vi "LSMcontroller_v59_PIzstage.vi"() -> ()   [LabVIEW 2015] (continued)
                                }
                                frame 5..7 {
                                n2125 = Index Array(array=w5021, index=0) -> (element=w5022:T19)
                                n2126 = call "waveformparamsv2.vi"("command"="get") -> ("Params out"=w5027:T15)  [unwired: 4 in, 2 out]
                                n2127 = in-place {
                                in-place-border: w5024 -> [w5031]
                                in-place-border: w5022 -> [w5029]
                                n2128 = in-place-cluster #43(w5027) -> ("DO parameters"=w5032:T18)
                                n2129 = in-place {
                                in-place-border: w5029 -> [w5033]
                                n2130 = in-place-array #44(w5032, w5031) -> ()  [unwired: 1 out]
                                n2131 = in-place-array #44(w5033) -> (w5030:T18)  [unwired: 1 out]
                                }
                                n2132 = in-place-cluster #43("DO parameters"=w5030) -> (w5025:T15)
                                }
                                n2133 = call "waveformparamsv2.vi"("command"="set", "Params in"=w5025) -> ()  [unwired: 3 in, 3 out]
                                }
                                }
                                }
                                frame #2 {
                                n2134 = local read "Measurement"() -> (w5035:T4)
                                n2135 = To Unsigned Long Integer(number=w5035) -> (unsigned 32bit integer=w5034:u32)
                                n2136 = case shown="5..7" w5034 {
                                tunnel: w5037 -> [_ w5041]
                                tunnel: w5036 -> [_ w5039]
                                frame 0..4, Default {
                                }
                                frame 5..7 {
                                n2137 = Index Array(array=w5039, index=0) -> (element=w5038:digitalwaveform)
                                n2138 = call "waveformsDObuffer.vi"("command"="get") -> ("DO wf out"=w5043:digitalwaveform[])  [unwired: 1 in]
                                n2139 = Replace Array Subset(array=w5043, new element=w5038, index=w5041) -> (w5045:digitalwaveform[])
                                n2140 = call "waveformsDObuffer.vi"("DO wf in"=w5045, "command"="set") -> ()  [unwired: 1 out]
                                }
                                }
                                }
                                }
                                }
                                }
                              }
                              frame #4 {
                                n2141 = call "Used AO lines.vi"() -> ("used AO names"=w5048:string[], "used AO lines"=w5046:tag[])  [unwired: 2 in]
                                n2142 = control-ref of="Analog Lines Plot"() -> (w5047:refnum<vi>)
                                n2143 = control-ref of="Digital Lines Plot"() -> (w5049:refnum<vi>)
                                n2144 = call "Used DO lines.vi"() -> ("used DO names"=w5050:string[], "used DO lines"=w5051:tag[])  [unwired: 2 in]
                                n2145 = local write "Analog Used Lines"(w5046) -> ()
                                n2146 = local write "Analog Used Names"(w5048) -> ()
                                n2147 = local write "Digital Used Lines"(w5051) -> ()
                                n2148 = local write "Digital Used Names"(w5050) -> ()
                                n2149 = call "prepDOWaveplot.vi"("DigitalGraph in"=w5049, "used DO names"=w5050) -> ()  [unwired: 1 in]
                                n2150 = call "prepAOWaveplot.vi"("WaveformGraph in"=w5047, "Analog Used Names"=w5048) -> ()  [unwired: 1 in]
                              }
                              frame #5 {
                                n2151 = local read "Meastab"() -> (w5066:enum32{"X-Y Image", "Linescan", "Timetrace"})
                                n2152 = property on="refwf" class="Ring (strict)"() -> ("RingText.Text"=w5063:string)  [unwired: 2 in, 2 out]
                                n2153 = case shown="\"Timetrace\"" w5066 {
                                tunnel: [w5068 w5069] -> w5067
                                frame "X-Y Image", Default {
                                n2154 = local read "Sampling rate"() -> (w5068:dbl)
                                }
                                frame "Timetrace" {
                                n2155 = local read "srateAODOtt"() -> (w5069:dbl)
                                }
                                }
                                n2156 = call "waveformsAObuffer.vi"("command"="get") -> ("AO wf out"=w5054:waveform(dbl)[])  [unwired: 1 in]
                                n2157 = local read "wavdet"() -> (w5064:bool)
                                n2158 = call "waveformsDObuffer.vi"("command"="get") -> ("DO wf out"=w5058:digitalwaveform[])  [unwired: 1 in]
                                n2159 = call "correctwaveformsizetemp.vi"("new sampling frequency (Hz)"=w5067, "start"=FALSE, "reference waveforms to"=w5063, "Analog waveforms in"=w5054, "stop"=TRUE, "Digital waveforms in"=w5058) -> ("analog wf out"=w5060:waveform(dbl)[], "Digital wf out"=w5062:digitalwaveform[], "measpoints"=w5065:i32)
                                n2160 = local write "Analog Lines Plot"(w5060) -> ()
                                n2161 = call "GetNumCamFramesv2.vi"("Digital Waveform Graph"=w5062) -> ("Numeric"=w5061:i32)  [unwired: 10 in]
                                n2162 = local write "Digital Lines Plot"(w5062) -> ()
                                n2163 = call "waveformsDObuffer.vi"("DO wf in"=w5062, "command"="set") -> ()  [unwired: 1 out]
                                n2164 = call "waveformsAObuffer.vi"("AO wf in"=w5060, "command"="set") -> ()  [unwired: 1 out]
                                n2165 = local write "Total Camera Frames"(w5061) -> ()
                                n2166 = case shown="True" w5064 {
                                tunnel: w5065 -> [_ w5070]
                                frame False {
                                }
                                frame True {
                                n2167 = local write "# of frames"(w5070) -> ()
                                }
                                }
                              }
                            }
                            n2168 = call "stoperaseCI.vi"() -> ()  [unwired: 12 in]
                            n2169 = call "stoperaseDO_img.vi"() -> ()  [unwired: 12 in]
                            n2170 = call "stoperaseAO_img.vi"() -> ()  [unwired: 12 in]
                            n2171 = call "stoperaseAI_img.vi"() -> ()  [unwired: 12 in]
                          }
                          frame #9 {
                            w5080 = FALSE ("Value (Signaling)")
                            n2172 = local read "save\ndata"() -> (w5075:bool)
                            n2173 = case shown="True" w5075 {
                              tunnel: w5074 -> [_ w5087]
                              frame False {
                              }
                              frame True {
                                n2174 = call "closebinaryfiles.vi"() -> ()  [unwired: 12 in]
                                n2175 = local read "filename prefix"() -> (w5089:string)
                                n2176 = local read "data dir"() -> (w5088:path)
                                n2177 = call "saveparams.vi"("timestamp"=w5087, "filename prefix in"=w5089, "data dir in"=w5088) -> ()  [unwired: 1 in]
                              }
                            }
                            n2178 = call "2pparameters.vi"("command"="get") -> ("params out"=w5071:T11)  [unwired: 1 in]
                            n2179 = Unbundle By Name(w5071) -> ("auto OD"=w5072:bool)
                            n2180 = case shown="True" w5072 {
                              frame False {
                              }
                              frame True {
                                n2181 = call "configuration.vi"("command"="get") -> ("config out"=w5083:T12)  [unwired: 2 in, 1 out]
                                n2182 = call "2pparameters.vi"("command"="get") -> ("params out"=w5086:T11)  [unwired: 1 in]
                                n2183 = Unbundle By Name(w5083) -> ("contour OD"=w5081:u16)
                                n2184 = Unbundle By Name(w5086) -> ("ODfilt"=w5082:u16)
                                n2185 = call "filterwheelcontrol_nothorlabslib.vi"("Current OD filt"=w5081, "New ODfilt"=w5082) -> ()  [unwired: 1 in]
                              }
                            }
                            n2186 = property on="Start" class="Bool (strict)"("Val(Sgnl)"=w5080) -> ()  [unwired: 2 in, 2 out]
                            n2187 = property on="Start" class="Bool (strict)"("Visible"=TRUE, "DisabledEnum"=T7."Enabled" ("Disabled")) -> ()  [unwired: 2 in, 2 out]
                            n2188 = property on="Stop" class="Bool (strict)"("Val(Sgnl)"=w5080) -> ()  [unwired: 2 in, 2 out]
                            n2189 = property on="Stop" class="Bool (strict)"("Visible"=FALSE, "DisabledEnum"=T7."Disabled" ("Disabled")) -> ()  [unwired: 2 in, 2 out]
                          }
                          frame #10 {
                            w5092 = T22 2 items=["no dialog", "OK message", "continue or stop message", "OK message + warnings", "continue/stop + warnings"] ("type of dialog (OK msg:1)")
                            n2190 = call "displayerrors.vi"() -> ("error IO"=w5093:errorcluster)
                            n2191 = call <vilib>:"General Error Handler.vi"("type of dialog (OK msg:1)"=w5092, "error in (no error)"=w5093) -> ("error out"=w5091:errorcluster)  [unwired: 9 in, 4 out]
                            n2192 = call <vilib>:"Clear Errors.vi"("error in (no error)"=w5091) -> ("error out"=w5090:errorcluster)  [unwired: 5 in, 1 out]
                            n2193 = call "seterrors.vi"("error IO"=w5090) -> ()
                          }
                        }
                      }
                    }
                  }
                  frame "Lifetime (point)" {
                    # "Disabled for conversion to 64 bit"
                    n2194 = disable-structure shown="Disabled" {
                      frame Disabled {
                        n2195 = stacked-sequence {
                          frame #0 {
                            w5104 = 12.5 ("x")
                            # "get from syncrate"
                            n2196 = local read "Bin size"() -> (w5098:T6)
                            n2197 = local read "Vx-ref"() -> (w5110:dbl)
                            n2198 = local read "Vy-ref"() -> (w5111:dbl)
                            n2199 = call "2pparameters.vi"("command"="get") -> ("params out"=w5096:T11)  [unwired: 1 in]
                            n2200 = Scale By Power Of 2(n=w5098, x=1.0 ("Y Scale.Range:Minimum")) -> (x*2^n=w5107:dbl)
                            n2201 = call "setposition.vi"("Vy"=w5111, "Vx"=w5110) -> ()  [unwired: 1 in]
                            n2202 = Unbundle By Name(w5096) -> ("autoshutter"=w5097:bool)
                            n2203 = Multiply(x=3000.0 ("Y Scale.Range:Minimum"), y=w5107) -> (x*y=w5105:dbl)
                            n2204 = Compound Arithmetic op=MULTIPLY(w5104, invert 3200.0 ("X Scale.Offset and Multiplier:Multiplier"), w5107) -> (w5106:dbl)
                            n2205 = case shown="True" w5097 {
                              frame False {
                              }
                              frame True {
                                n2206 = call "shuttercontrol.vi"("command"="open") -> ()  [unwired: 1 in, 1 out]
                              }
                            }
                            n2207 = call "lifetimeparameters.vi"("command"="get") -> ("Params out"=w5102:T20)  [unwired: 1 in]
                            n2208 = property on="Histogram" class="WFGraph (strict)"("XScale.Maximum"=w5104, "XScale.Minimum"=0.0 ("X Scale.Range:Minimum"), "YScale.Maximum"=w5105, "YScale.Minimum"=0.1 ("Y Scale.Range:Minimum"), "XScale.Multiplier"=w5106) -> ()  [unwired: 2 in, 2 out]
                            n2209 = Bundle By Name(cluster=w5102, "Bin size"=w5098) -> (w5103:T20)
                            n2210 = call "lifetimeparameters.vi"("Params in"=w5103, "command"="set") -> ()  [unwired: 1 out]
                            n2211 = property on="Histogram 2" class="WFGraph (strict)"("YScale.Maximum"=w5105, "XScale.Multiplier"=w5106, "XScale.Maximum"=w5104) -> ()  [unwired: 2 in, 2 out]
                            n2212 = call "2pparameters.vi"("command"="get") -> ("params out"=w5118:T11)  [unwired: 1 in]
                            n2213 = Bundle By Name(cluster=w5118, "type"="Lifetime (point)") -> (w5116:T11)
                            n2214 = property on="Stop" class="Bool (strict)"("Visible"=TRUE, "DisabledEnum"=T7."Enabled" ("Disabled")) -> ()  [unwired: 2 in, 2 out]
                            n2215 = property on="Start" class="Bool (strict)"("Visible"=FALSE, "DisabledEnum"=T7."Disabled and Grayed Out" ("Disabled")) -> ()  [unwired: 2 in, 2 out]
                            n2216 = call "2pparameters.vi"("Params in"=w5116, "command"="set") -> ()  [unwired: 1 out]
                          }
                          frame #1 {
                            n2217 = call "setup.vi"() -> ()  [unwired: 1 in]
                          }
                          frame #2 {
                            # "main loop"
                            n2218 = call "lifetimeparameters.vi"("command"="get") -> ("Params out"=w5128:T20)  [unwired: 1 in]
                            n2219 = Unbundle By Name(w5128) -> ("devidx"=w5126:i32)
                            n2220 = for {
                              N: 10000 -> [_]
                              tunnel: [w5129] -> w5124 mode=indexing
                              i -> [w5129]
                            }
                            n2221 = while {
                              tunnel: w5126 -> [w5133]
                              tunnel: w5124 -> [w5130]
                              i -> [w5131]
                              stop <- w5135 stop-if-true
                              n2222 = Increment(x=w5131) -> (x+1=w5132:i32)
                              n2223 = dll-call lib="phlib.dll" fn="_PH_GetCountRate@8" label="PH_GetCountRate"("devidx"=w5133, "channel"=0) -> (w5134:i32)  [unwired: 5 in, 2 out]
                              "SyncRate" <- w5134
                              n2224 = stacked-sequence {
                                seq-local: [_ _ w5142 _ _] -> [_ _ _ w5155 _]
                                seq-local: [_ _ w5141 _ _] -> [_ _ _ w5154 _]
                                seq-local: [_ w5139 _ _ _] -> [_ _ w5143 _ _]
                                tunnel: w5134 -> [_ _ _ w5162 _]
                                tunnel: w5130 -> [_ _ _ w5152 _]
                                frame #0 {
                                n2225 = call "start_binned.vi"() -> ()  [unwired: 1 in]
                                }
                                frame #1 {
                                n2226 = call "get-histogram.vi"() -> ("IntegralCount"=→"Integral count":u32, "Histogram"=w5139:u32[])
                                "Histogram" <- w5139
                                }
                                frame #2 {
                                n2227 = Search 1D Array(1D array=w5143, element=u32 0) -> (index of element=w5141:i32)  [unwired: 1 in]
                                n2228 = Multiply(x=w5141, y=0.99) -> (x*y=w5147:dbl)
                                n2229 = Array Subset(array=w5143, index=0, length=w5147) -> (w5150:u32[])
                                n2230 = Array Max & Min(array=w5150) -> (max index (indices)=w5144:i32)  [unwired: 3 out]
                                n2231 = Split 1D Array(array=w5150, index=w5144) -> (second subarray=w5146:u32[])  [unwired: 1 out]
                                n2232 = Array Max & Min(array=w5146) -> (min index (indices)=w5145:i32)  [unwired: 3 out]
                                n2233 = Split 1D Array(array=w5146, index=w5145) -> (first subarray=w5142:u32[])  [unwired: 1 out]
                                "Histogram 2" <- w5142
                                }
                                frame #3 {
                                n2234 = Array Size(array=w5155) -> (size(s)=w5157:i32)
                                n2235 = Array Subset(array=w5152, index=0, length=w5157) -> (w5156:i32[])
                                n2236 = Compound Arithmetic op=MULTIPLY(1000000000.0 ("value"), invert w5162, invert w5154, w5156) -> (w5153:dbl[])
                                n2237 = call <vilib>:"Exponential Fit.vi"("Y"=w5155, "X"=w5153) -> ("damping"=w5159:dbl)  [unwired: 8 in, 5 out]
                                n2238 = Divide(x=-1.0 ("y"), y=w5159) -> (x/y=→"Lifetime (ns)":dbl)
                                }
                                frame #4 {
                                n2239 = local read "downright"() -> (w5169:bool)
                                n2240 = local read "downleft"() -> (w5171:bool)
                                n2241 = local read "upright"() -> (w5167:bool)
                                n2242 = local read "upleft"() -> (w5165:bool)
                                n2243 = local read "down"() -> (w5170:bool)
                                n2244 = local read "right"() -> (w5168:bool)
                                n2245 = local read "left"() -> (w5172:bool)
                                n2246 = local read "up"() -> (w5166:bool)
                                n2247 = Compound Arithmetic op=OR(w5165, w5166, w5167, w5168, w5169, w5170, w5171, w5172) -> (w5164:bool)
                                n2248 = case shown="True" w5164 {
                                frame False {
                                }
                                frame True {
                                n2249 = stacked-sequence {
                                frame #0 {
                                n2250 = local read "downright"() -> (w5174:bool)
                                n2251 = local read "downleft"() -> (w5176:bool)
                                n2252 = local read "BigSmall"() -> (w5173:bool)
                                n2253 = local read "upright"() -> (w5178:bool)
                                n2254 = local read "upleft"() -> (w5181:bool)
                                n2255 = local read "down"() -> (w5177:bool)
                                n2256 = local read "right"() -> (w5179:bool)
                                n2257 = local read "left"() -> (w5175:bool)
                                n2258 = local read "up"() -> (w5180:bool)
                                n2259 = call "movestageparams.vi"("command"="get") -> ("Params out"=w5184:T21)  [unwired: 1 in]
                                n2260 = Bundle By Name(cluster=w5184, "upleft"=w5181, "up"=w5180, "upright"=w5178, "right"=w5179, "downright"=w5174, "down"=w5177, "downleft"=w5176, "left"=w5175, "Bigsmall"=w5173) -> (w5185:T21)
                                n2261 = call "movestageparams.vi"("Params in"=w5185, "command"="set") -> ()  [unwired: 1 out]
                                }
                                frame #1 {
                                n2262 = call "movestage.vi"() -> ()  [unwired: 12 in]
                                }
                                frame #2 {
                                w5186 = FALSE ("OK Button")
                                w5187 = FALSE ("OK Button")
                                n2263 = property on="down" class="Bool (strict)"("Value"=w5187) -> ()  [unwired: 2 in, 2 out]
                                n2264 = property on="up" class="Bool (strict)"("Value"=w5187) -> ()  [unwired: 2 in, 2 out]
                                n2265 = property on="right" class="Bool (strict)"("Value"=w5187) -> ()  [unwired: 2 in, 2 out]
                                n2266 = property on="left" class="Bool (strict)"("Value"=w5187) -> ()  [unwired: 2 in, 2 out]
                                n2267 = property on="upleft" class="Bool (strict)"("Value"=w5186) -> ()  [unwired: 2 in, 2 out]
                                n2268 = property on="upright" class="Bool (strict)"("Value"=w5186) -> ()  [unwired: 2 in, 2 out]
                                n2269 = property on="downleft" class="Bool (strict)"("Value"=w5186) -> ()  [unwired: 2 in, 2 out]
                                n2270 = property on="downright" class="Bool (strict)"("Value"=w5186) -> ()  [unwired: 2 in, 2 out]
                                }
                                }
                                }
                                }
                                }
                              }
                              n2271 = dll-call lib="phlib.dll" fn="_PH_GetCountRate@8" label="PH_GetCountRate"("devidx"=w5133, "channel"=1) -> (→"Ch1Rate":i32)  [unwired: 5 in, 2 out]
                              n2272 = local read "Stop"() -> (w5135:bool)
                              n2273 = local write "points recorded"(w5132) -> ()
                            }
                          }
                          frame #3 {
                            w5195 = FALSE ("Value (Signaling)")
                            n2274 = call "2pparameters.vi"("command"="get") -> ("params out"=w5189:T11)  [unwired: 1 in]
                            n2275 = Unbundle By Name(w5189) -> ("autoshutter"=w5190:bool)
                            n2276 = case shown="True" w5190 {
                              frame False {
                              }
                              frame True {
                                n2277 = call "shuttercontrol.vi"("command"="close") -> ()  [unwired: 1 in, 1 out]
                              }
                            }
                            n2278 = property on="Start" class="Bool (strict)"("Val(Sgnl)"=w5195) -> ()  [unwired: 2 in, 2 out]
                            n2279 = property on="Start" class="Bool (strict)"("Visible"=TRUE, "DisabledEnum"=T7."Enabled" ("Disabled")) -> ()  [unwired: 2 in, 2 out]
                            n2280 = property on="Stop" class="Bool (strict)"("Val(Sgnl)"=w5195) -> ()  [unwired: 2 in, 2 out]
                            n2281 = property on="Stop" class="Bool (strict)"("Visible"=FALSE, "DisabledEnum"=T7."Disabled" ("Disabled")) -> ()  [unwired: 2 in, 2 out]
                          }
                        }
                      }
                      frame Enabled {
                      }
                    }
                    n2282 = local write "64bit disabled"(TRUE ("64bit disabled")) -> ()
                  }
                }
              }
            }
          }
          event "avpp", "Angle ref", "xpixels ref", "Vx-min ref", "Vx-max ref", "ypixels ref", "Vy-min ref", "Vy-max ref", "ROI Type", "Sampling rate": Value Change {
            n2283 = event-data() -> ()  [unwired: 1 in, 6 out]
            n2284 = local read "avpp"() -> (w5214:i32)
            n2285 = local read "Angle ref"() -> (w5213:dbl)
            n2286 = local read "ROI Type"() -> (w5212:u16)
            n2287 = local read "xpixels ref"() -> (w5209:i32)
            n2288 = local read "Vx-min ref"() -> (w5208:dbl)
            n2289 = local read "Vx-max ref"() -> (w5207:dbl)
            n2290 = local read "ypixels ref"() -> (w5205:i32)
            n2291 = local read "Vy-min ref"() -> (w5206:dbl)
            n2292 = local read "Vy-max ref"() -> (w5202:dbl)
            n2293 = local read "Sampling rate"() -> (w5197:dbl)
            n2294 = local read "# of frames"() -> (w5201:i32)
            n2295 = local read "maxbufferAI"() -> (w5200:i32)
            n2296 = local read "Override AI buffer"() -> (w5198:bool)
            n2297 = call "2pparameters.vi"("command"="get") -> ("params out"=w5211:T11)  [unwired: 1 in]
            n2298 = Bundle By Name(cluster=w5211, "avpp"=w5214, "Angle Img"=w5213, "Xpixels Img"=w5209, "Vx-min Img"=w5208, "VX-max Img"=w5207, "Ypixels Img"=w5205, "Vy-min Img"=w5206, "Vy-max Img"=w5202, "srate"=w5197, "srate Img"=w5197, "measpoints"=w5201, "maxbufferAI"=w5200, "Drawing Mode"=w5212, "Vz-reset"=0.0, "AIoverride"=w5198) -> (w5203:T11)
            n2299 = call "2pparameters.vi"("Params in"=w5203, "command"="set") -> ()  [unwired: 1 out]
          }
          event "# of frames": Value Change {
            n2300 = event-data() -> ()  [unwired: 1 in, 6 out]
            n2301 = local read "Meastab"() -> (w5215:enum32{"X-Y Image", "Linescan", "Timetrace"})
            n2302 = case shown="\"X-Y Image\", Default" w5215 {
              frame "X-Y Image", Default {
                n2303 = local read "# of frames"() -> (w5216:i32)
                n2304 = call "2pparameters.vi"("command"="get") -> ("params out"=w5220:T11)  [unwired: 1 in]
                n2305 = Bundle By Name(cluster=w5220, "measpoints"=w5216) -> (w5217:T11)
                n2306 = call "2pparameters.vi"("Params in"=w5217, "command"="set") -> ()  [unwired: 1 out]
              }
              frame "Linescan" {
                n2307 = local read "srateAODOtt"() -> (w5230:dbl)
                n2308 = local read "# of frames"() -> (w5226:i32)
                n2309 = local read "refreshtime"() -> (w5232:dbl)
                n2310 = local read "bin"() -> (w5227:dbl)
                n2311 = call "tt_timeandsamples.vi"("bin"=w5227, "refreshtime"=w5232, "srateAODOtt"=w5230, "tot#ofsamples"=w5226) -> ("refreshrate"=w5229:dbl, "refreshbuffer"=w5228:i32, "timetracecycles"=w5225:i32)  [unwired: 5 in]
                n2312 = call "2pparameters.vi"("command"="get") -> ("params out"=w5222:T11)  [unwired: 1 in]
                n2313 = Bundle By Name(cluster=w5222, "measpoints"=w5226, "tt_cycles"=w5225, "refreshbuffer"=w5228, "refreshrate"=w5229) -> (w5224:T11)
                n2314 = Reciprocal(x=w5229) -> (1/x=w5231:dbl)
                n2315 = local write "refreshtime"(w5231) -> ()
                n2316 = call "2pparameters.vi"("Params in"=w5224, "command"="set") -> ()  [unwired: 1 out]
              }
              frame "Timetrace" {
                n2317 = local read "srateAODOtt"() -> (w5242:dbl)
                n2318 = local read "# of frames"() -> (w5238:i32)
                n2319 = local read "refreshtime"() -> (w5244:dbl)
                n2320 = local read "bin"() -> (w5239:dbl)
                n2321 = call "tt_timeandsamples.vi"("bin"=w5239, "refreshtime"=w5244, "srateAODOtt"=w5242, "tot#ofsamples"=w5238) -> ("refreshrate"=w5241:dbl, "refreshbuffer"=w5240:i32, "timetracecycles"=w5237:i32)  [unwired: 5 in]
                n2322 = call "2pparameters.vi"("command"="get") -> ("params out"=w5234:T11)  [unwired: 1 in]
                n2323 = Bundle By Name(cluster=w5234, "measpoints"=w5238, "tt_cycles"=w5237, "refreshbuffer"=w5240, "refreshrate"=w5241) -> (w5236:T11)
                n2324 = Reciprocal(x=w5241) -> (1/x=w5243:dbl)
                n2325 = local write "refreshtime"(w5243) -> ()
                n2326 = call "2pparameters.vi"("Params in"=w5236, "command"="set") -> ()  [unwired: 1 out]
              }
            }
          }
          event "srateAODOtt", "refreshtime", "Vx-ref", "Vy-ref", "Vx-min draw", "Vx-max draw", "Vy-min draw", "Vy-max draw", "bin": Value Change {
            n2327 = event-data() -> ()  [unwired: 1 in, 6 out]
            n2328 = local read "ypixels ref"() -> (w5276:i32)
            n2329 = local read "Vy-min draw"() -> (w5252:dbl)
            n2330 = local read "Vy-max draw"() -> (w5251:dbl)
            n2331 = local read "Vx-min draw"() -> (w5254:dbl)
            n2332 = local read "Vx-max draw"() -> (w5253:dbl)
            n2333 = local read "xpixels ref"() -> (w5250:i32)
            n2334 = local read "ROI Type"() -> (w5249:u16)
            n2335 = local read "Pel"() -> (w5248:dbl)
            n2336 = local read "srateAODOtt"() -> (w5258:dbl)
            n2337 = local read "# of frames"() -> (w5263:i32)
            n2338 = local read "refreshtime"() -> (w5256:dbl)
            n2339 = local read "bin"() -> (w5261:dbl)
            n2340 = local read "Override AI buffer"() -> (w5246:bool)
            n2341 = local read "finite samples"() -> (w5270:bool)
            n2342 = local read "srateAODOtt"() -> (w5245:dbl)
            n2343 = local read "srateAODOtt"() -> (w5264:dbl)
            n2344 = local read "continuous"() -> (w5269:bool)
            n2345 = local read "Angle ref"() -> (w5255:dbl)
            n2346 = local read "wavdet"() -> (w5271:bool)
            n2347 = local read "Vx-ref"() -> (w5266:dbl)
            n2348 = local read "Vy-ref"() -> (w5268:dbl)
            n2349 = local read "avpp"() -> (w5267:i32)
            n2350 = call "tt_timeandsamples.vi"("bin"=w5261, "refreshtime"=w5256, "srateAODOtt"=w5258, "tot#ofsamples"=w5263) -> ("refreshrate"=w5259:dbl, "refreshbuffer"=w5260:i32, "timetracecycles"=w5265:i32)  [unwired: 5 in]
            n2351 = local read "bin"() -> (w5262:dbl)
            n2352 = call "2pparameters.vi"("command"="get") -> ("params out"=w5274:T11)  [unwired: 1 in]
            n2353 = Bundle By Name(cluster=w5274, "Drawing Mode"=w5249, "measpoints"=w5263, "tt_cycles"=w5265, "refreshbuffer"=w5260, "refreshrate"=w5259, "Vx-ref"=w5266, "Vy-ref"=w5268, "srate"=w5245, "finite"=w5270, "cont"=w5269, "wavdet"=w5271, "avpp"=w5267, "srateAODO"=w5264, "bufferAI"=w5260, "bin"=w5262, "Angle Img"=w5255, "Vxminref"=w5254, "Vxmaxref"=w5253, "Vyminref"=w5252, "Vymaxref"=w5251, "Xpixels Img"=w5250, "Ypixels Img"=w5276, "Pel"=w5248, "Vz-reset"=0.0, "AIoverride"=w5246) -> (w5272:T11)
            n2354 = Reciprocal(x=w5259) -> (1/x=w5257:dbl)
            n2355 = local write "refreshtime"(w5257) -> ()
            n2356 = call "2pparameters.vi"("Params in"=w5272, "command"="set") -> ()  [unwired: 1 out]
          }
          event "Init": Value Change {
            # "Disabled for conversion to 64 bit"
            n2357 = event-data() -> ()  [unwired: 1 in, 6 out]
            n2358 = disable-structure shown="Disabled" {
              frame Disabled {
                n2359 = flat-sequence {
                  frame #0 {
                    n2360 = local read "Measurement"() -> (w5278:T4)
                    n2361 = case shown="\"Lifetime (scan)\", \"Lifetime (contour)\"" w5278 {
                      frame "X-Y-t movie", Default {
                      }
                      frame "Lifetime (point)" {
                        n2362 = stacked-sequence {
                          frame #0 {
                            n2363 = call "initialize.vi"("mode"=0) -> ()
                          }
                          frame #1 {
                            n2364 = call "calib.vi"() -> ()  [unwired: 1 in]
                          }
                        }
                      }
                      frame "Lifetime (scan)", "Lifetime (contour)" {
                        n2365 = stacked-sequence {
                          frame #0 {
                            n2366 = call "initialize.vi"("mode"=3) -> ()
                          }
                          frame #1 {
                            n2367 = call "calib.vi"() -> ()  [unwired: 1 in]
                          }
                        }
                      }
                    }
                  }
                  frame #1 {
                    n2368 = property on="Start" class="Bool (strict)"("Visible"=TRUE, "DisabledEnum"=T7."Enabled" ("Disabled")) -> ()  [unwired: 2 in, 2 out]
                    n2369 = property on="Init" class="Bool (strict)"("Visible"=FALSE, "DisabledEnum"=T7."Disabled and Grayed Out" ("Disabled"), "Value"=FALSE ("Init")) -> ()  [unwired: 2 in, 2 out]
                  }
                }
              }
              frame Enabled {
              }
            }
            n2370 = local write "64bit disabled"(TRUE ("64bit disabled")) -> ()
          }
          event "Measurement": Value Change {
            n2371 = event-data() -> ()  [unwired: 1 in, 5 out]
            n2372 = case shown="\"Lifetime (contour)\"" "Measurement" {
              frame "X-Y-t movie" {
                w5288 = T7."Disabled" ("Disabled")
                w5287 = FALSE ("Visible")
                n2373 = call "2pparameters.vi"("command"="get") -> ("params out"=w5298:T11)  [unwired: 1 in]
                n2374 = local write "graphtab"(T5."image" ("graphtab")) -> ()
                n2375 = local write "Save tab"(enum32{"withsave", "withoutsave"}."withsave" ("Save tab")) -> ()
                n2376 = Bundle By Name(cluster=w5298, "type"="X-Y-t movie") -> (w5296:T11)
                n2377 = call "2pparameters.vi"("Params in"=w5296, "command"="set") -> ()  [unwired: 1 out]
                n2378 = property on="refreshtime" class="DigNum (strict)"("Visible"=FALSE, "DisabledEnum"=T7."Disabled and Grayed Out" ("Disabled")) -> ()  [unwired: 2 in, 2 out]
                n2379 = property on="ttt" class="Enum (strict)"("Visible"=FALSE) -> ()  [unwired: 2 in, 2 out]
                n2380 = property on="# of frames" class="DigNum (strict)"("DisabledEnum"=T7."Enabled" ("Disabled"), "Caption.Text"="# of frames") -> ()  [unwired: 2 in, 2 out]
                n2381 = property on="continuous" class="Bool (strict)"("Visible"=TRUE, "DisabledEnum"=T7."Enabled" ("Disabled")) -> ()  [unwired: 2 in, 2 out]
                n2382 = property on="finite samples" class="Bool (strict)"("Visible"=TRUE, "DisabledEnum"=T7."Enabled" ("Disabled")) -> ()  [unwired: 2 in, 2 out]
                n2383 = property on="avpp" class="DigNum (strict)"("Visible"=TRUE, "DisabledEnum"=T7."Enabled" ("Disabled")) -> ()  [unwired: 2 in, 2 out]
                n2384 = property on="srateAODOtt" class="DigNum (strict)"("Visible"=FALSE, "DisabledEnum"=T7."Disabled" ("Disabled")) -> ()  [unwired: 2 in, 2 out]
                n2385 = local write "save\ndata"(TRUE ("save\ndata")) -> ()
                n2386 = property on="finite samples" class="Bool (strict)"("Val(Sgnl)"=TRUE ("continuous for display")) -> ()  [unwired: 2 in, 2 out]
                n2387 = property on="continuous" class="Bool (strict)"("Value"=FALSE ("continuous for display")) -> ()  [unwired: 2 in, 2 out]
                n2388 = property on="Current Average" class="DigNum (strict)"("Visible"=TRUE, "DisabledEnum"=T7."Enabled" ("Disabled")) -> ()  [unwired: 2 in, 2 out]
                n2389 = property on="img_CH1" class="IntGraph (strict)"("ZScale.Maximum"=7.0 ("Z Scale.Range:Maximum")) -> ()  [unwired: 2 in, 2 out]
                n2390 = property on="Sampling rate" class="DigNum (strict)"("Visible"=TRUE, "DisabledEnum"=T7."Enabled" ("Disabled")) -> ()  [unwired: 2 in, 2 out]
                n2391 = property on="Pel" class="DigNum (strict)"("Visible"=w5287, "DisabledEnum"=w5288) -> ()  [unwired: 2 in, 2 out]
                n2392 = property on="bin" class="DigNum (strict)"("Visible"=w5287, "DisabledEnum"=w5288) -> ()  [unwired: 2 in, 2 out]
                "Meastab" <- enum32{"X-Y Image", "Linescan", "Timetrace"}."X-Y Image" ("Meastab")
                "Zscantab" <- enum32{"withzscan", "withoutzscan", "lifetime"}."withoutzscan" ("Zscantab")
              }
              frame "X-Y-Z stack" {
                w5320 = T7."Disabled" ("Disabled")
                w5319 = FALSE ("Visible")
                n2393 = call "2pparameters.vi"("command"="get") -> ("params out"=w5330:T11)  [unwired: 1 in]
                n2394 = call "2pparameters.vi"("command"="get") -> ("params out"=w5334:T11)  [unwired: 1 in]
                n2395 = Bundle By Name(cluster=w5330, "type"="X-Y-Z stack") -> (w5328:T11)
                n2396 = Unbundle By Name(w5334) -> ("motorref"=w5333:refnum<k7>)
                n2397 = call "2pparameters.vi"("Params in"=w5328, "command"="set") -> ()  [unwired: 1 out]
                n2398 = local write "Zscantab"(enum32{"withzscan", "withoutzscan", "lifetime"}."withzscan" ("Zscantab")) -> ()
                n2399 = local write "Meastab"(enum32{"X-Y Image", "Linescan", "Timetrace"}."X-Y Image" ("Meastab")) -> ()
                n2400 = invoke class="MG17Motor" method="GetPosition"(reference=w5333, "lChanID"=0, "pfPosition"=sgl 0.0) -> ("pfPosition"=w5345:sgl)  [unwired: 2 in, 4 out]
                n2401 = property on="refreshtime" class="DigNum (strict)"("Visible"=FALSE, "DisabledEnum"=T7."Disabled and Grayed Out" ("Disabled")) -> ()  [unwired: 2 in, 2 out]
                n2402 = property on="ttt" class="Enum (strict)"("Visible"=FALSE) -> ()  [unwired: 2 in, 2 out]
                n2403 = Multiply(x=w5345, y=1000.0) -> (x*y=w5344:dbl)
                n2404 = local write "Actual Z position"(w5344) -> ()
                n2405 = local write "Save tab"(enum32{"withsave", "withoutsave"}."withsave" ("Save tab")) -> ()
                n2406 = property on="finite samples" class="Bool (strict)"("Visible"=FALSE, "DisabledEnum"=T7."Disabled and Grayed Out" ("Disabled")) -> ()  [unwired: 2 in, 2 out]
                n2407 = property on="avpp" class="DigNum (strict)"("Visible"=TRUE, "DisabledEnum"=T7."Enabled" ("Disabled")) -> ()  [unwired: 2 in, 2 out]
                n2408 = property on="continuous" class="Bool (strict)"("Visible"=FALSE, "DisabledEnum"=T7."Disabled and Grayed Out" ("Disabled")) -> ()  [unwired: 2 in, 2 out]
                n2409 = property on="img_CH1" class="IntGraph (strict)"("ZScale.Maximum"=7.0 ("Z Scale.Range:Maximum")) -> ()  [unwired: 2 in, 2 out]
                n2410 = property on="srateAODOtt" class="DigNum (strict)"("Visible"=FALSE, "DisabledEnum"=T7."Disabled" ("Disabled")) -> ()  [unwired: 2 in, 2 out]
                n2411 = property on="Pel" class="DigNum (strict)"("Visible"=w5319, "DisabledEnum"=w5320) -> ()  [unwired: 2 in, 2 out]
                n2412 = property on="bin" class="DigNum (strict)"("Visible"=w5319, "DisabledEnum"=w5320) -> ()  [unwired: 2 in, 2 out]
                n2413 = property on="Current Average" class="DigNum (strict)"("Visible"=TRUE, "DisabledEnum"=T7."Enabled" ("Disabled")) -> ()  [unwired: 2 in, 2 out]
                n2414 = property on="# of frames" class="DigNum (strict)"("Caption.Text"="# of slices", "DisabledEnum"=T7."Disabled and Grayed Out" ("Disabled")) -> ()  [unwired: 2 in, 2 out]
                n2415 = local write "save\ndata"(TRUE ("save\ndata")) -> ()
                n2416 = property on="finite samples" class="Bool (strict)"("Val(Sgnl)"=TRUE ("continuous for display")) -> ()  [unwired: 2 in, 2 out]
                n2417 = property on="continuous" class="Bool (strict)"("Value"=FALSE ("continuous for display")) -> ()  [unwired: 2 in, 2 out]
                n2418 = property on="Sampling rate" class="DigNum (strict)"("Visible"=TRUE, "DisabledEnum"=T7."Enabled" ("Disabled")) -> ()  [unwired: 2 in, 2 out]
              }
              frame "X-Y-Z-t movie" {
                w5359 = T7."Disabled" ("Disabled")
                w5358 = FALSE ("Visible")
                n2419 = property on="# of frames" class="DigNum (strict)"("DisabledEnum"=T7."Enabled" ("Disabled")) -> ()  [unwired: 2 in, 2 out]
                n2420 = property on="Current Average" class="DigNum (strict)"("Visible"=TRUE, "DisabledEnum"=T7."Enabled" ("Disabled")) -> ()  [unwired: 2 in, 2 out]
                n2421 = property on="avpp" class="DigNum (strict)"("Visible"=TRUE, "DisabledEnum"=T7."Enabled" ("Disabled")) -> ()  [unwired: 2 in, 2 out]
                n2422 = local write "Save tab"(enum32{"withsave", "withoutsave"}."withsave" ("Save tab")) -> ()
                n2423 = local write "Zscantab"(enum32{"withzscan", "withoutzscan", "lifetime"}."withzscan" ("Zscantab")) -> ()
                n2424 = local write "Meastab"(enum32{"X-Y Image", "Linescan", "Timetrace"}."X-Y Image" ("Meastab")) -> ()
                n2425 = property on="refreshtime" class="DigNum (strict)"("Visible"=FALSE, "DisabledEnum"=T7."Disabled and Grayed Out" ("Disabled")) -> ()  [unwired: 2 in, 2 out]
                n2426 = property on="ttt" class="Enum (strict)"("Visible"=FALSE) -> ()  [unwired: 2 in, 2 out]
                n2427 = call "2pparameters.vi"("command"="get") -> ("params out"=w5369:T11)  [unwired: 1 in]
                n2428 = Bundle By Name(cluster=w5369, "type"="X-Y-Z-t movie") -> (w5367:T11)
                n2429 = property on="continuous" class="Bool (strict)"("Visible"=TRUE, "DisabledEnum"=T7."Enabled" ("Disabled")) -> ()  [unwired: 2 in, 2 out]
                n2430 = property on="finite samples" class="Bool (strict)"("Visible"=TRUE, "DisabledEnum"=T7."Enabled" ("Disabled")) -> ()  [unwired: 2 in, 2 out]
                n2431 = call "2pparameters.vi"("Params in"=w5367, "command"="set") -> ()  [unwired: 1 out]
                n2432 = property on="srateAODOtt" class="DigNum (strict)"("Visible"=FALSE, "DisabledEnum"=T7."Disabled" ("Disabled")) -> ()  [unwired: 2 in, 2 out]
                n2433 = local write "save\ndata"(TRUE ("save\ndata")) -> ()
                n2434 = property on="img_CH1" class="IntGraph (strict)"("ZScale.Maximum"=7.0 ("Z Scale.Range:Maximum")) -> ()  [unwired: 2 in, 2 out]
                n2435 = property on="continuous" class="Bool (strict)"("Value"=FALSE ("continuous for display")) -> ()  [unwired: 2 in, 2 out]
                n2436 = property on="finite samples" class="Bool (strict)"("Value"=TRUE ("continuous for display")) -> ()  [unwired: 2 in, 2 out]
                n2437 = property on="Sampling rate" class="DigNum (strict)"("Visible"=TRUE, "DisabledEnum"=T7."Enabled" ("Disabled")) -> ()  [unwired: 2 in, 2 out]
                n2438 = property on="Pel" class="DigNum (strict)"("Visible"=w5358, "DisabledEnum"=w5359) -> ()  [unwired: 2 in, 2 out]
                n2439 = property on="bin" class="DigNum (strict)"("Visible"=w5358, "DisabledEnum"=w5359) -> ()  [unwired: 2 in, 2 out]
              }
              frame "linescan" {
                w5389 = T7."Enabled" ("Disabled")
                w5388 = TRUE ("Visible")
                w5391 = T7."Enabled" ("Disabled")
                w5390 = TRUE ("Visible")
                n2440 = local write "Meastab"(enum32{"X-Y Image", "Linescan", "Timetrace"}."Linescan" ("Meastab")) -> ()
                n2441 = property on="Current Average" class="DigNum (strict)"("Visible"=TRUE, "DisabledEnum"=T7."Enabled" ("Disabled")) -> ()  [unwired: 2 in, 2 out]
                n2442 = local write "Save tab"(enum32{"withsave", "withoutsave"}."withsave" ("Save tab")) -> ()
                n2443 = local write "Zscantab"(enum32{"withzscan", "withoutzscan", "lifetime"}."withoutzscan" ("Zscantab")) -> ()
                n2444 = property on="refreshtime" class="DigNum (strict)"("Visible"=FALSE, "DisabledEnum"=T7."Disabled and Grayed Out" ("Disabled")) -> ()  [unwired: 2 in, 2 out]
                n2445 = property on="continuous" class="Bool (strict)"("Value"=FALSE ("continuous for display")) -> ()  [unwired: 2 in, 2 out]
                n2446 = property on="finite samples" class="Bool (strict)"("Value"=TRUE ("continuous for display")) -> ()  [unwired: 2 in, 2 out]
                n2447 = property on="ttt" class="Enum (strict)"("Visible"=FALSE) -> ()  [unwired: 2 in, 2 out]
                n2448 = local write "save\ndata"(TRUE ("save\ndata")) -> ()
                n2449 = call "2pparameters.vi"("command"="get") -> ("params out"=w5400:T11)  [unwired: 1 in]
                n2450 = Bundle By Name(cluster=w5400, "type"="linescan") -> (w5398:T11)
                n2451 = property on="# of frames" class="DigNum (strict)"("DisabledEnum"=T7."Enabled" ("Disabled"), "Caption.Text"="# of lines") -> ()  [unwired: 2 in, 2 out]
                n2452 = property on="continuous" class="Bool (strict)"("Visible"=TRUE, "DisabledEnum"=T7."Enabled" ("Disabled")) -> ()  [unwired: 2 in, 2 out]
                n2453 = property on="avpp" class="DigNum (strict)"("Visible"=TRUE, "DisabledEnum"=T7."Enabled" ("Disabled")) -> ()  [unwired: 2 in, 2 out]
                n2454 = property on="finite samples" class="Bool (strict)"("Visible"=TRUE, "DisabledEnum"=T7."Enabled" ("Disabled")) -> ()  [unwired: 2 in, 2 out]
                n2455 = property on="srateAODOtt" class="DigNum (strict)"("Visible"=TRUE, "DisabledEnum"=T7."Enabled" ("Disabled")) -> ()  [unwired: 2 in, 2 out]
                n2456 = call "2pparameters.vi"("Params in"=w5398, "command"="set") -> ()  [unwired: 1 out]
                n2457 = property on="Pel" class="DigNum (strict)"("Visible"=w5390, "DisabledEnum"=w5391) -> ()  [unwired: 2 in, 2 out]
                n2458 = property on="bin" class="DigNum (strict)"("Visible"=w5390, "DisabledEnum"=w5391) -> ()  [unwired: 2 in, 2 out]
                n2459 = property on="Sampling rate" class="DigNum (strict)"("Visible"=FALSE, "DisabledEnum"=T7."Disabled" ("Disabled")) -> ()  [unwired: 2 in, 2 out]
                n2460 = property on="Pel" class="DigNum (strict)"("Visible"=w5388, "DisabledEnum"=w5389) -> ()  [unwired: 2 in, 2 out]
                n2461 = property on="bin" class="DigNum (strict)"("Visible"=w5388, "DisabledEnum"=w5389) -> ()  [unwired: 2 in, 2 out]
              }
              frame "Timetrace" {
                w5421 = T7."Enabled" ("Disabled")
                w5420 = TRUE ("Visible")
                n2462 = call "2pparameters.vi"("command"="get") -> ("params out"=w5426:T11)  [unwired: 1 in]
                n2463 = local write "Meastab"(enum32{"X-Y Image", "Linescan", "Timetrace"}."Timetrace" ("Meastab")) -> ()
                n2464 = Unbundle By Name(w5426) -> ("Angle draw"=w5428:dbl)
                n2465 = local write "Zscantab"(enum32{"withzscan", "withoutzscan", "lifetime"}."withoutzscan" ("Zscantab")) -> ()
                n2466 = property on="# of frames" class="DigNum (strict)"("DisabledEnum"=T7."Enabled" ("Disabled"), "Caption.Text"="# of samples") -> ()  [unwired: 2 in, 2 out]
                n2467 = property on="refreshtime" class="DigNum (strict)"("Visible"=TRUE, "DisabledEnum"=T7."Enabled" ("Disabled")) -> ()  [unwired: 2 in, 2 out]
                n2468 = property on="avpp" class="DigNum (strict)"("Visible"=FALSE, "DisabledEnum"=T7."Disabled and Grayed Out" ("Disabled")) -> ()  [unwired: 2 in, 2 out]
                n2469 = property on="Current Average" class="DigNum (strict)"("Visible"=FALSE, "DisabledEnum"=T7."Disabled and Grayed Out" ("Disabled")) -> ()  [unwired: 2 in, 2 out]
                n2470 = local write "Angle drawing"(w5428) -> ()
                n2471 = property on="ttt" class="Enum (strict)"("Visible"=TRUE) -> ()  [unwired: 2 in, 2 out]
                n2472 = property on="continuous" class="Bool (strict)"("Visible"=TRUE, "DisabledEnum"=T7."Enabled" ("Disabled")) -> ()  [unwired: 2 in, 2 out]
                n2473 = property on="finite samples" class="Bool (strict)"("Visible"=TRUE, "DisabledEnum"=T7."Enabled" ("Disabled")) -> ()  [unwired: 2 in, 2 out]
                n2474 = local write "save\ndata"(TRUE ("save\ndata")) -> ()
                n2475 = property on="finite samples" class="Bool (strict)"("Val(Sgnl)"=TRUE ("continuous for display")) -> ()  [unwired: 2 in, 2 out]
                n2476 = property on="continuous" class="Bool (strict)"("Value"=FALSE ("continuous for display")) -> ()  [unwired: 2 in, 2 out]
                n2477 = local write "Save tab"(enum32{"withsave", "withoutsave"}."withsave" ("Save tab")) -> ()
                n2478 = property on="srateAODOtt" class="DigNum (strict)"("Visible"=TRUE, "DisabledEnum"=T7."Enabled" ("Disabled")) -> ()  [unwired: 2 in, 2 out]
                n2479 = call "2pparameters.vi"("command"="get") -> ("params out"=w5433:T11)  [unwired: 1 in]
                n2480 = Bundle By Name(cluster=w5433, "type"="Timetrace") -> (w5431:T11)
                n2481 = property on="Sampling rate" class="DigNum (strict)"("Visible"=FALSE, "DisabledEnum"=T7."Disabled" ("Disabled")) -> ()  [unwired: 2 in, 2 out]
                n2482 = property on="Pel" class="DigNum (strict)"("Visible"=w5420, "DisabledEnum"=w5421) -> ()  [unwired: 2 in, 2 out]
                n2483 = property on="bin" class="DigNum (strict)"("Visible"=w5420, "DisabledEnum"=w5421) -> ()  [unwired: 2 in, 2 out]
                n2484 = call "2pparameters.vi"("Params in"=w5431, "command"="set") -> ()  [unwired: 1 out]
              }
              frame "Lifetime (point)" {
                w5454 = T7."Enabled" ("Disabled")
                w5453 = TRUE ("Visible")
                n2485 = property on="Pel" class="DigNum (strict)"("Visible"=w5453, "DisabledEnum"=w5454) -> ()  [unwired: 2 in, 2 out]
                n2486 = property on="bin" class="DigNum (strict)"("Visible"=w5453, "DisabledEnum"=w5454) -> ()  [unwired: 2 in, 2 out]
                n2487 = property on="ttt" class="Enum (strict)"("Visible"=FALSE) -> ()  [unwired: 2 in, 2 out]
                n2488 = local write "Zscantab"(enum32{"withzscan", "withoutzscan", "lifetime"}."lifetime" ("Zscantab")) -> ()
                n2489 = local write "graphtab"(T5."Lifetime" ("graphtab")) -> ()
                n2490 = local write "Meastab"(enum32{"X-Y Image", "Linescan", "Timetrace"}."Timetrace" ("Meastab")) -> ()
                n2491 = call "lifetimeparameters.vi"("command"="get") -> ("Params out"=w5461:T20)  [unwired: 1 in]
                n2492 = Unbundle By Name(w5461) -> ("initialized"=w5462:bool)
                n2493 = property on="srateAODOtt" class="DigNum (strict)"("Visible"=TRUE, "DisabledEnum"=T7."Enabled" ("Disabled")) -> ()  [unwired: 2 in, 2 out]
                n2494 = case shown="False" w5462 {
                  frame False {
                    n2495 = property on="Init" class="Bool (strict)"("Visible"=TRUE, "DisabledEnum"=T7."Enabled" ("Disabled")) -> ()  [unwired: 2 in, 2 out]
                    n2496 = property on="Start" class="Bool (strict)"("Visible"=FALSE, "DisabledEnum"=T7."Disabled and Grayed Out" ("Disabled")) -> ()  [unwired: 2 in, 2 out]
                  }
                  frame True {
                  }
                }
                n2497 = property on="Sampling rate" class="DigNum (strict)"("Visible"=FALSE, "DisabledEnum"=T7."Disabled" ("Disabled")) -> ()  [unwired: 2 in, 2 out]
              }
              frame "Lifetime (scan)" {
                w5471 = T7."Disabled" ("Disabled")
                w5470 = FALSE ("Visible")
                n2498 = call "lifetimeparameters.vi"("command"="get") -> ("Params out"=w5483:T20)  [unwired: 1 in]
                n2499 = local write "graphtab"(T5."image" ("graphtab")) -> ()
                n2500 = local write "Save tab"(enum32{"withsave", "withoutsave"}."withsave" ("Save tab")) -> ()
                n2501 = local write "Meastab"(enum32{"X-Y Image", "Linescan", "Timetrace"}."X-Y Image" ("Meastab")) -> ()
                n2502 = local write "Zscantab"(enum32{"withzscan", "withoutzscan", "lifetime"}."lifetime" ("Zscantab")) -> ()
                n2503 = Unbundle By Name(w5483) -> ("initialized"=w5482:bool)
                n2504 = property on="ttt" class="Enum (strict)"("Visible"=FALSE) -> ()  [unwired: 2 in, 2 out]
                n2505 = property on="refreshtime" class="DigNum (strict)"("Visible"=FALSE, "DisabledEnum"=T7."Disabled and Grayed Out" ("Disabled")) -> ()  [unwired: 2 in, 2 out]
                n2506 = property on="Pel" class="DigNum (strict)"("Visible"=w5470, "DisabledEnum"=w5471) -> ()  [unwired: 2 in, 2 out]
                n2507 = property on="bin" class="DigNum (strict)"("Visible"=w5470, "DisabledEnum"=w5471) -> ()  [unwired: 2 in, 2 out]
                n2508 = property on="save data" class="Bool (strict)"("Visible"=TRUE, "DisabledEnum"=T7."Enabled" ("Disabled"), "Value"=TRUE ("Visible")) -> ()  [unwired: 2 in, 2 out]
                n2509 = case shown="False" w5482 {
                  frame False {
                    n2510 = property on="Init" class="Bool (strict)"("Visible"=TRUE, "DisabledEnum"=T7."Enabled" ("Disabled")) -> ()  [unwired: 2 in, 2 out]
                    n2511 = property on="Start" class="Bool (strict)"("Visible"=FALSE, "DisabledEnum"=T7."Disabled and Grayed Out" ("Disabled")) -> ()  [unwired: 2 in, 2 out]
                  }
                  frame True {
                  }
                }
                n2512 = call "2pparameters.vi"("command"="get") -> ("params out"=w5488:T11)  [unwired: 1 in]
                n2513 = property on="continuous" class="Bool (strict)"("Visible"=TRUE, "DisabledEnum"=T7."Disabled and Grayed Out" ("Disabled")) -> ()  [unwired: 2 in, 2 out]
                n2514 = property on="finite samples" class="Bool (strict)"("Visible"=TRUE, "DisabledEnum"=T7."Enabled" ("Disabled")) -> ()  [unwired: 2 in, 2 out]
                n2515 = Bundle By Name(cluster=w5488, "type"="Lifetime (scan)") -> (w5486:T11)
                n2516 = call "2pparameters.vi"("Params in"=w5486, "command"="set") -> ()  [unwired: 1 out]
                n2517 = property on="finite samples" class="Bool (strict)"("Val(Sgnl)"=TRUE ("continuous for display")) -> ()  [unwired: 2 in, 2 out]
                n2518 = property on="continuous" class="Bool (strict)"("Value"=FALSE ("continuous for display")) -> ()  [unwired: 2 in, 2 out]
                n2519 = property on="srateAODOtt" class="DigNum (strict)"("Visible"=FALSE, "DisabledEnum"=T7."Disabled" ("Disabled")) -> ()  [unwired: 2 in, 2 out]
                n2520 = property on="# of frames" class="DigNum (strict)"("DisabledEnum"=T7."Enabled" ("Disabled"), "Caption.Text"="# of frames") -> ()  [unwired: 2 in, 2 out]
                n2521 = property on="img_CH1" class="IntGraph (strict)"("ZScale.Maximum"=12.5 ("Z Scale.Range:Maximum")) -> ()  [unwired: 2 in, 2 out]
                n2522 = property on="Current Average" class="DigNum (strict)"("Visible"=TRUE, "DisabledEnum"=T7."Enabled" ("Disabled")) -> ()  [unwired: 2 in, 2 out]
                n2523 = property on="Sampling rate" class="DigNum (strict)"("Visible"=TRUE, "DisabledEnum"=T7."Enabled" ("Disabled")) -> ()  [unwired: 2 in, 2 out]
                n2524 = property on="avpp" class="DigNum (strict)"("Visible"=TRUE, "DisabledEnum"=T7."Enabled" ("Disabled")) -> ()  [unwired: 2 in, 2 out]
              }
              frame "Lifetime (contour)" {
                w5512 = T7."Enabled" ("Disabled")
                w5511 = TRUE ("Visible")
                n2525 = call "2pparameters.vi"("command"="get") -> ("params out"=w5519:T11)  [unwired: 1 in]
                n2526 = property on="# of frames" class="DigNum (strict)"("DisabledEnum"=T7."Enabled" ("Disabled"), "Caption.Text"="# of samples") -> ()  [unwired: 2 in, 2 out]
                n2527 = property on="refreshtime" class="DigNum (strict)"("Visible"=TRUE, "DisabledEnum"=T7."Enabled" ("Disabled")) -> ()  [unwired: 2 in, 2 out]
                n2528 = Unbundle By Name(w5519) -> ("Angle draw"=w5521:dbl)
                n2529 = property on="avpp" class="DigNum (strict)"("Visible"=FALSE, "DisabledEnum"=T7."Disabled and Grayed Out" ("Disabled")) -> ()  [unwired: 2 in, 2 out]
                n2530 = property on="Current Average" class="DigNum (strict)"("Visible"=FALSE, "DisabledEnum"=T7."Disabled and Grayed Out" ("Disabled")) -> ()  [unwired: 2 in, 2 out]
                n2531 = local write "Angle drawing"(w5521) -> ()
                n2532 = local write "Save tab"(enum32{"withsave", "withoutsave"}."withsave" ("Save tab")) -> ()
                n2533 = local write "Zscantab"(enum32{"withzscan", "withoutzscan", "lifetime"}."lifetime" ("Zscantab")) -> ()
                n2534 = local write "graphtab"(T5."Lifetime" ("graphtab")) -> ()
                n2535 = local write "Meastab"(enum32{"X-Y Image", "Linescan", "Timetrace"}."Timetrace" ("Meastab")) -> ()
                n2536 = property on="ttt" class="Enum (strict)"("Visible"=TRUE) -> ()  [unwired: 2 in, 2 out]
                n2537 = call "lifetimeparameters.vi"("command"="get") -> ("Params out"=w5543:T20)  [unwired: 1 in]
                n2538 = property on="finite samples" class="Bool (strict)"("Val(Sgnl)"=TRUE ("continuous for display")) -> ()  [unwired: 2 in, 2 out]
                n2539 = local write "save\ndata"(TRUE ("save\ndata")) -> ()
                n2540 = Unbundle By Name(w5543) -> ("initialized"=w5544:bool)
                n2541 = property on="continuous" class="Bool (strict)"("Visible"=TRUE, "DisabledEnum"=T7."Enabled" ("Disabled")) -> ()  [unwired: 2 in, 2 out]
                n2542 = property on="finite samples" class="Bool (strict)"("Visible"=TRUE, "DisabledEnum"=T7."Enabled" ("Disabled")) -> ()  [unwired: 2 in, 2 out]
                n2543 = property on="Pel" class="DigNum (strict)"("Visible"=w5511, "DisabledEnum"=w5512) -> ()  [unwired: 2 in, 2 out]
                n2544 = property on="bin" class="DigNum (strict)"("Visible"=w5511, "DisabledEnum"=w5512) -> ()  [unwired: 2 in, 2 out]
                n2545 = property on="continuous" class="Bool (strict)"("Value"=FALSE ("continuous for display")) -> ()  [unwired: 2 in, 2 out]
                n2546 = case shown="False" w5544 {
                  frame False {
                    n2547 = property on="Init" class="Bool (strict)"("Visible"=TRUE, "DisabledEnum"=T7."Enabled" ("Disabled")) -> ()  [unwired: 2 in, 2 out]
                    n2548 = property on="Start" class="Bool (strict)"("Visible"=FALSE, "DisabledEnum"=T7."Disabled and Grayed Out" ("Disabled")) -> ()  [unwired: 2 in, 2 out]
                  }
                  frame True {
                  }
                }
                n2549 = property on="srateAODOtt" class="DigNum (strict)"("Visible"=TRUE, "DisabledEnum"=T7."Enabled" ("Disabled")) -> ()  [unwired: 2 in, 2 out]
                n2550 = call "2pparameters.vi"("command"="get") -> ("params out"=w5523:T11)  [unwired: 1 in]
                n2551 = Bundle By Name(cluster=w5523, "type"="Timetrace") -> (w5517:T11)
                n2552 = call "2pparameters.vi"("Params in"=w5517, "command"="set") -> ()  [unwired: 1 out]
                n2553 = property on="Sampling rate" class="DigNum (strict)"("Visible"=FALSE, "DisabledEnum"=T7."Disabled" ("Disabled")) -> ()  [unwired: 2 in, 2 out]
              }
            }
          }
          event "Laserpower \n(%)": Value Change {
            n2554 = event-data() -> ("OldVal"=w5552:dbl, "NewVal"=w5553:dbl)  [unwired: 1 in, 4 out]
            n2555 = Not Equal?(x=w5552, y=w5553) -> (x != y?=w5554:bool)
            n2556 = case shown="True" w5554 {
              tunnel: w5553 -> [_ w5555]
              frame False {
              }
              frame True {
                n2557 = local read "wavelength(nm)"() -> (w5557:dbl)
                n2558 = call "configuration.vi"("command"="get") -> ("config out"=w5561:T12)  [unwired: 2 in, 1 out]
                n2559 = call "pockelscellcalibration.vi"("l"=w5557, "T"=w5555) -> ("Vout"=w5556:dbl)
                n2560 = Unbundle By Name(w5561) -> ("Vto2P"=w5560:i32, "AOlines"=w5559:tag[])
                n2561 = property on="lpow" class="DigNum (strict)"("Value"=w5555) -> ()  [unwired: 2 in, 2 out]
                n2562 = Index Array(array=w5559, index=w5560) -> (element=w5558:tag)
                n2563 = call-poly <vilib>:"DAQmx Create Virtual Channel.vi"("physical channels"=w5558) -> ("task out"=w5564:refnum<k21>, "error out"=w5563:errorcluster)  [unwired: 13 in]
                n2564 = call-poly <vilib>:"DAQmx Write.vi"("task/channels in"=w5564, "data"=w5556, "error in"=w5563) -> ("task out"=w5565:refnum<k21>, "error out"=w5566:errorcluster)  [unwired: 10 in, 1 out]
                n2565 = call <vilib>:"DAQmx Start Task.vi"("task/channels in"=w5565, "error in"=w5566) -> ("task out"=w5567:refnum<k21>, "error out"=w5568:errorcluster)  [unwired: 12 in]
                n2566 = call <vilib>:"DAQmx Stop Task.vi"("task/channels in"=w5567, "error in"=w5568) -> ("task out"=w5569:refnum<k21>, "error out"=w5570:errorcluster)  [unwired: 12 in]
                n2567 = call <vilib>:"DAQmx Clear Task.vi"("task in"=w5569, "error in"=w5570) -> ()  [unwired: 13 in, 1 out]
              }
            }
          }
          event "lpow": Value Change {
            n2568 = event-data() -> ("OldVal"=w5571:dbl, "NewVal"=w5572:dbl)  [unwired: 1 in, 4 out]
            n2569 = Not Equal?(x=w5571, y=w5572) -> (x != y?=w5573:bool)
            n2570 = case shown="True" w5573 {
              tunnel: w5572 -> [_ w5576]
              frame False {
              }
              frame True {
                n2571 = local read "wavelength(nm)"() -> (w5575:dbl)
                n2572 = call "pockelscellcalibration.vi"("l"=w5575, "T"=w5576) -> ("Vout"=w5574:dbl)
                n2573 = call "configuration.vi"("command"="get") -> ("config out"=w5580:T12)  [unwired: 2 in, 1 out]
                n2574 = Unbundle By Name(w5580) -> ("Vto2P"=w5579:i32, "AOlines"=w5578:tag[])
                n2575 = property on="Laserpower \n(%)" class="Slide (strict)"("Value"=w5576) -> ()  [unwired: 2 in, 2 out]
                n2576 = Index Array(array=w5578, index=w5579) -> (element=w5577:tag)
                n2577 = call-poly <vilib>:"DAQmx Create Virtual Channel.vi"("physical channels"=w5577) -> ("task out"=w5583:refnum<k21>, "error out"=w5582:errorcluster)  [unwired: 13 in]
                n2578 = call-poly <vilib>:"DAQmx Write.vi"("task/channels in"=w5583, "data"=w5574, "error in"=w5582) -> ("task out"=w5584:refnum<k21>, "error out"=w5585:errorcluster)  [unwired: 10 in, 1 out]
                n2579 = call <vilib>:"DAQmx Start Task.vi"("task/channels in"=w5584, "error in"=w5585) -> ("task out"=w5586:refnum<k21>, "error out"=w5587:errorcluster)  [unwired: 12 in]
                n2580 = call <vilib>:"DAQmx Stop Task.vi"("task/channels in"=w5586, "error in"=w5587) -> ("task out"=w5588:refnum<k21>, "error out"=w5589:errorcluster)  [unwired: 12 in]
                n2581 = call <vilib>:"DAQmx Clear Task.vi"("task in"=w5588, "error in"=w5589) -> ()  [unwired: 13 in, 1 out]
              }
            }
          }
          event "sealtest": Value Change {
            n2582 = event-data() -> ()  [unwired: 1 in, 6 out]
            n2583 = case shown="True" "sealtest" {
              frame False {
              }
              frame True {
                n2584 = stacked-sequence {
                  seq-local: [w5591 _ _ _ _ _] -> [_ w5624 _ w5676 _ _]
                  frame #0 {
                    n2585 = stacked-sequence {
                      tunnel: [_ w5603 _] -> w5591
                      frame #0 {
                        n2586 = call "2pparameters.vi"("command"="get") -> ("params out"=w5596:T11)  [unwired: 1 in]
                        n2587 = Unbundle By Name(w5596) -> ("autoshutter"=w5597:bool)
                        n2588 = local read "OCchecked?"() -> (w5594:bool)
                        n2589 = call "sealtestwfparams.vi"("command"="set") -> ()  [unwired: 6 in, 1 out]
                        n2590 = case shown="False" w5594 {
                          frame False {
                            n2591 = One Button Dialog(message="Is the OC gain correct?", button name ("OK")="ok") -> (true=w5598:bool)
                            n2592 = local write "OCchecked?"(w5598) -> ()
                          }
                          frame True {
                          }
                        }
                        n2593 = case shown="True" w5597 {
                          frame False {
                          }
                          frame True {
                            n2594 = call "shuttercontrol.vi"("command"="close") -> ()  [unwired: 1 in, 1 out]
                          }
                        }
                        n2595 = call "allAI-temp.vi"("command"=enum16{"get", "set", "clear", "append"}."clear") -> ()  [unwired: 3 in, 2 out]
                      }
                      frame #1 {
                        n2596 = call "sealtestwfparams.vi"("command"="get") -> ("Params out"=w5609:T24)  [unwired: 6 in]
